vi "test_read-nmea-data2.vi"() -> ()   [LabVIEW 2019] (continued)
\t\n15:11:41.31\tF9P\t$GNGSA,A,3,12,06,19,05,17,09,04,02,,,,,1.44,0.74,1.23,1*02\n\t\n15:11:41.33\tF9P\t$GNGSA,A,3,85,71,84,,,,,,,,,,1.44,0.74,1.23,2*07\n\t\n15:11:41.35\tF9P\t$GNGSA,A,3,36,19,11,04,09,12,,,,,,,1.44,0.74,1.23,3*02\n\t\n15:11:41.37\tF9P\t$GNGSA,A,3,14,11,33,,,,,,,,,,1.44,0.74,1.23,4*03\n\t\n15:11:41.39\tF9P\t$GPGSV,3,1,09,02,54,318,23,04,18,044,22,05,37,247,25,06,64,047,32,1*6B\n\t\n15:11:41.41\tF9P\t$GPGSV,3,2,09,09,45,074,35,12,24,277,34,17,33,153,35,19,53,157,30,1*68\n\t\n15:11:41.43\tF9P\t$GPGSV,3,3,09,25,12,307,20,1*5F\n\t\n15:11:41.45\tF9P\t$GPGSV,3,1,09,02,54,318,,04,18,044,17,05,37,247,,06,64,047,23,6*6C\n\t\n15:11:41.47\tF9P\t$GPGSV,3,2,09,09,45,074,26,12,24,277,23,17,33,153,27,19,53,157,,6*6B\n\t\n15:11:41.49\tF9P\t$GPGSV,3,3,09,25,12,307,,6*5A\n\t\n15:11:41.51\tF9P\t$GLGSV,2,1,08,69,12,031,,70,71,039,,71,52,205,35,72,04,209,,1*7C\n\t\n15:11:41.53\tF9P\t$GLGSV,2,2,08,77,01,326,,84,20,122,13,85,70,065,30,86,36,330,,1*7A\n\t\n15:11:41.55\tF9P\t$GLGSV,2,1,08,69,12,031,,70,71,039,,71,52,205,25,72,04,209,,3*7F\n\t\n15:11:41.57\tF9P\t$GLGSV,2,2,08,77,01,326,,84,20,122,18,85,70,065,22,86,36,330,,3*70\n\t\n15:11:41.59\tF9P\t$GAGSV,2,1,08,02,08,297,07,04,66,118,29,09,32,193,29,11,71,358,26,7*7A\n\t\n15:11:41.61\tF9P\t$GAGSV,2,2,08,12,40,102,28,19,26,045,22,25,09,249,,36,26,308,35,7*75\n\t\n15:11:41.63\tF9P\t$GAGSV,2,1,08,02,08,297,,04,66,118,34,09,32,193,,11,71,358,,2*7B\n\t\n15:11:41.65\tF9P\t$GAGSV,2,2,08,12,40,102,,19,26,045,,25,09,249,,36,26,308,,2*7C\n\t\n15:11:41.67\tF9P\t$GBGSV,1,1,03,11,50,132,26,14,87,127,26,33,60,219,28,1*48\n\t\n15:11:41.69\tF9P\t$GBGSV,1,1,03,11,50,132,33,14,87,127,,33,60,219,,3*40\n\t\n15:11:41.71\tF9P\t$GNGLL,3723.52576,N,12656.91469,E,061143.00,A,A*75\n\t\n15:11:41.73\tF9P\t\t\n15:11:41.75\tF9P\t\t\n15:11:41.77\tF9P\t\t\n15:11:41.79\tF9P\t\t\n15:11:41.81\tF9P\t\t\n15:11:41.83\tF9P\t\t\n15:11:41.85\tF9P\t\t\n15:11:41.87\tF9P\t\t\n15:11:41.89\tF9P\t\t\n15:11:41.91\tF9P\t\t\n15:11:41.93\tF9P\t\t\n15:11:41.95\tF9P\t\t\n15:11:41.97\tF9P\t\t\n15:11:41.99\tF9P\t\t\n15:11:42.01\tF9P\t\t\n15:11:42.03\tF9P\t\t\n15:11:42.05\tF9P\t\t\n15:11:42.07\tF9P\t\t\n15:11:42.09\tF9P\t\t\n15:11:42.11\tF9P\t\t\n15:11:42.13\tF9P\t\t\n15:11:42.15\tF9P\t\t\n15:11:42.17\tF9P\t\t\n15:11:42.19\tF9P\t\t\n15:11:42.21\tF9P\t\t\n15:11:42.23\tF9P\t\t\n15:11:42.25\tF9P\t$GNRMC,061144.00,A,3723.52558,N,12656.91506,E,1.761,99.51,250720,,,A,V*3C\n\t\n15:11:42.27\tF9P\t$GNVTG,99.51,T,,M,1.761,N,3.262,K,A*13\n\t\n15:11:42.29\tF9P\t$GNGGA,061144.00,3723.52558,N,12656.91506,E,1,12,0.71,35.1,M,18.5,M,,*7D\n\t\n15:11:42.31\tF9P\t$GNGSA,A,3,12,06,19,05,17,09,04,02,,,,,1.29,0.71,1.08,1*05\n\t\n15:11:42.33\tF9P\t$GNGSA,A,3,85,71,84,,,,,,,,,,1.29,0.71,1.08,2*00\n\t\n15:11:42.35\tF9P\t$GNGSA,A,3,36,19,11,04,09,12,,,,,,,1.29,0.71,1.08,3*05\n\t\n15:11:42.37\tF9P\t$GNGSA,A,3,14,11,33,,,,,,,,,,1.29,0.71,1.08,4*04\n\t\n15:11:42.39\tF9P\t$GPGSV,3,1,09,02,54,318,26,04,18,044,22,05,37,247,25,06,64,047,31,1*6D\n\t\n15:11:42.41\tF9P\t$GPGSV,3,2,09,09,45,074,34,12,24,277,42,17,33,153,32,19,53,157,30,1*6F\n\t\n15:11:42.43\tF9P\t$GPGSV,3,3,09,25,12,307,21,1*5E\n\t\n15:11:42.45\tF9P\t$GPGSV,3,1,09,02,54,318,,04,18,044,17,05,37,247,,06,64,047,31,6*6F\n\t\n15:11:42.47\tF9P\t$GPGSV,3,2,09,09,45,074,31,12,24,277,25,17,33,153,26,19,53,157,,6*6A\n\t\n15:11:42.49\tF9P\t$GPGSV,3,3,09,25,12,307,,6*5A\n\t\n15:11:42.51\tF9P\t$GLGSV,2,1,08,69,12,031,,70,71,039,,71,52,205,37,72,04,209,,1*7E\n\t\n15:11:42.53\tF9P\t$GLGSV,2,2,08,77,01,326,,84,20,122,09,85,70,065,31,86,36,330,,1*70\n\t\n15:11:42.55\tF9P\t$GLGSV,2,1,08,69,12,031,,70,71,039,,71,52,205,26,72,04,209,,3*7C\n\t\n15:11:42.57\tF9P\t$GLGSV,2,2,08,77,01,326,,84,20,122,19,85,70,065,29,86,36,330,,3*7A\n\t\n15:11:42.59\tF9P\t$GAGSV,2,1,08,02,08,297,14,04,66,118,29,09,32,193,29,11,71,358,31,7*7E\n\t\n15:11:42.61\tF9P\t$GAGSV,2,2,08,12,40,102,32,19,26,045,22,25,09,249,,36,26,308,32,7*79\n\t\n15:11:42.63\tF9P\t$GAGSV,2,1,08,02,08,297,,04,66,118,33,09,32,193,,11,71,358,,2*7C\n\t\n15:11:42.65\tF9P\t$GAGSV,2,2,08,12,40,102,,19,26,045,,25,09,249,,36,26,308,,2*7C\n\t\n15:11:42.67\tF9P\t$GBGSV,1,1,03,11,50,132,28,14,87,127,26,33,60,219,36,1*49\n\t\n15:11:42.69\tF9P\t$GBGSV,1,1,03,11,50,132,33,14,87,127,,33,60,219,,3*40\n\t\n15:11:42.71\tF9P\t$GNGLL,3723.52558,N,12656.91506,E,061144.00,A,A*76\n\t\n15:11:42.73\tF9P\t\t\n15:11:42.75\tF9P\t\t\n15:11:42.77\tF9P\t\t\n15:11:42.79\tF9P\t\t\n15:11:42.81\tF9P\t\t\n15:11:42.83\tF9P\t\t\n15:11:42.85\tF9P\t\t\n15:11:42.87\tF9P\t\t\n15:11:42.89\tF9P\t\t\n15:11:42.91\tF9P\t\t\n15:11:42.93\tF9P\t\t\n15:11:42.95\tF9P\t\t\n15:11:42.97\tF9P\t\t\n15:11:42.99\tF9P\t\t\n15:11:43.01\tF9P\t\t\n15:11:43.03\tF9P\t\t\n15:11:43.05\tF9P\t\t\n15:11:43.07\tF9P\t\t\n15:11:43.09\tF9P\t\t\n15:11:43.11\tF9P\t\t\n15:11:43.13\tF9P\t\t\n15:11:43.15\tF9P\t\t\n15:11:43.17\tF9P\t\t\n15:11:43.19\tF9P\t\t\n15:11:43.21\tF9P\t\t\n15:11:43.23\tF9P\t\t\n15:11:43.25\tF9P\t$GNRMC,061145.00,A,3723.52534,N,12656.91513,E,1.259,108.79,250720,,,A,V*0E\n\t\n15:11:43.27\tF9P\t$GNVTG,108.79,T,,M,1.259,N,2.331,K,A*28\n\t\n15:11:43.29\tF9P\t$GNGGA,061145.00,3723.52534,N,12656.91513,E,1,12,0.71,36.9,M,18.5,M,,*79\n\t\n15:11:43.31\tF9P\t$GNGSA,A,3,12,06,19,05,17,09,04,02,,,,,1.29,0.71,1.08,1*05\n\t\n15:11:43.33\tF9P\t$GNGSA,A,3,85,71,84,,,,,,,,,,1.29,0.71,1.08,2*00\n\t\n15:11:43.35\tF9P\t$GNGSA,A,3,36,19,11,04,09,12,,,,,,,1.29,0.71,1.08,3*05\n\t\n15:11:43.37\tF9P\t$GNGSA,A,3,14,11,33,,,,,,,,,,1.29,0.71,1.08,4*04\n\t\n15:11:43.39\tF9P\t$GPGSV,3,1,09,02,54,318,34,04,18,044,22,05,37,247,25,06,64,047,27,1*69\n\t\n15:11:43.41\tF9P\t$GPGSV,3,2,09,09,45,074,36,12,24,277,42,17,33,153,38,19,53,157,29,1*6F\n\t\n15:11:43.43\tF9P\t$GPGSV,3,3,09,25,12,307,20,1*5F\n\t\n15:11:43.45\tF9P\t$GPGSV,3,1,09,02,54,318,,04,18,044,15,05,37,247,17,06,64,047,24,6*6F\n\t\n15:11:43.47\tF9P\t$GPGSV,3,2,09,09,45,074,28,12,24,277,31,17,33,153,23,19,53,157,,6*62\n\t\n15:11:43.49\tF9P\t$GPGSV,3,3,09,25,12,307,,6*5A\n\t\n15:11:43.51\tF9P\t$GLGSV,2,1,08,69,12,031,,70,71,039,,71,52,205,43,72,04,209,,1*7D\n\t\n15:11:43.53\tF9P\t$GLGSV,2,2,08,77,01,326,,84,20,122,11,85,70,065,37,86,36,330,,1*7F\n\t\n15:11:43.55\tF9P\t$GLGSV,2,1,08,69,12,031,,70,71,039,,71,52,205,25,72,04,209,,3*7F\n\t\n15:11:43.57\tF9P\t$GLGSV,2,2,08,77,01,326,,84,20,122,19,85,70,065,21,86,36,330,,3*72\n\t\n15:11:43.59\tF9P\t$GAGSV,2,1,08,02,08,297,09,04,66,118,29,09,32,193,34,11,71,358,34,7*7B\n\t\n15:11:43.61\tF9P\t$GAGSV,2,2,08,12,40,102,32,19,26,045,23,25,09,249,,36,26,308,35,7*7F\n\t\n15:11:43.63\tF9P\t$GAGSV,2,1,08,02,08,297,,04,66,118,,09,32,193,,11,71,358,,2*7C\n\t\n15:11:43.65\tF9P\t$GAGSV,2,2,08,12,40,102,,19,26,045,,25,09,249,,36,26,308,,2*7C\n\t\n15:11:43.67\tF9P\t$GBGSV,1,1,03,11,50,132,32,14,87,127,32,33,60,219,35,1*44\n\t\n15:11:43.69\tF9P\t$GBGSV,1,1,03,11,50,132,29,14,87,127,29,33,60,219,,3*40\n\t\n15:11:43.71\tF9P\t$GNGLL,3723.52534,N,12656.91513,E,061145.00,A,A*79\n\t\n15:11:43.73\tF9P\t\t\n15:11:43.75\tF9P\t\t\n15:11:43.77\tF9P\t\t\n15:11:43.79\tF9P\t\t\n15:11:43.81\tF9P\t\t\n15:11:43.83\tF9P\t\t\n15:11:43.85\tF9P\t\t\n15:11:43.87\tF9P\t\t\n15:11:43.89\tF9P\t\t\n15:11:43.91\tF9P\t\t\n15:11:43.93\tF9P\t\t\n15:11:43.95\tF9P\t\t\n15:11:43.97\tF9P\t\t\n15:11:43.99\tF9P\t\t\n15:11:44.01\tF9P\t\t\n15:11:44.03\tF9P\t\t\n15:11:44.05\tF9P\t\t\n15:11:44.07\tF9P\t\t\n15:11:44.09\tF9P\t\t\n15:11:44.11\tF9P\t\t\n15:11:44.13\tF9P\t\t\n15:11:44.15\tF9P\t\t\n15:11:44.17\tF9P\t\t\n15:11:44.19\tF9P\t\t\n15:11:44.21\tF9P\t\t\n15:11:44.23\tF9P\t\t\n15:11:44.25\tF9P\t$GNRMC,061146.00,A,3723.52516,N,12656.91546,E,1.741,93.31,250720,,,A,V*3E\n\t\n15:11:44.27\tF9P\t$GNVTG,93.31,T,,M,1.741,N,3.225,K,A*1E\n\t\n15:11:44.29\tF9P\t$GNGGA,061146.00,3723.52516,N,12656.91546,E,1,12,0.74,37.2,M,18.5,M,,*75\n\t\n15:11:44.31\tF9P\t$GNGSA,A,3,12,06,19,05,17,09,04,02,,,,,1.44,0.74,1.23,1*02\n\t\n15:11:44.33\tF9P\t$GNGSA,A,3,85,71,84,,,,,,,,,,1.44,0.74,1.23,2*07\n\t\n15:11:44.35\tF9P\t$GNGSA,A,3,36,19,11,04,09,12,,,,,,,1.44,0.74,1.23,3*02\n\t\n15:11:44.37\tF9P\t$GNGSA,A,3,14,11,33,,,,,,,,,,1.44,0.74,1.23,4*03\n\t\n15:11:44.39\tF9P\t$GPGSV,3,1,09,02,54,318,38,04,18,044,20,05,37,247,26,06,64,047,28,1*6B\n\t\n15:11:44.41\tF9P\t$GPGSV,3,2,09,09,45,074,37,12,24,277,42,17,33,153,35,19,53,157,35,1*6E\n\t\n15:11:44.43\tF9P\t$GPGSV,3,3,09,25,12,307,19,1*55\n\t\n15:11:44.45\tF9P\t$GPGSV,3,1,09,02,54,318,,04,18,044,15,05,37,247,16,06,64,047,22,6*68\n\t\n15:11:44.47\tF9P\t$GPGSV,3,2,09,09,45,074,26,12,24,277,26,17,33,153,23,19,53,157,,6*6A\n\t\n15:11:44.49\tF9P\t$GPGSV,3,3,09,25,12,307,,6*5A\n\t\n15:11:44.51\tF9P\t$GLGSV,2,1,08,69,12,031,,70,71,039,,71,52,205,40,72,04,209,,1*7E\n\t\n15:11:44.53\tF9P\t$GLGSV,2,2,08,77,01,326,,84,20,122,15,85,70,065,23,86,36,330,,1*7E\n\t\n15:11:44.55\tF9P\t$GLGSV,2,1,08,69,12,031,,70,71,039,,71,52,205,26,72,04,209,,3*7C\n\t\n15:11:44.57\tF9P\t$GLGSV,2,2,08,77,01,326,,84,20,122,20,85,70,065,29,86,36,330,,3*70\n\t\n15:11:44.59\tF9P\t$GAGSV,2,1,08,02,08,297,07,04,66,118,33,09,32,193,37,11,71,358,33,7*7A\n\t\n15:11:44.61\tF9P\t$GAGSV,2,2,08,12,40,102,36,19,26,045,21,25,09,249,,36,26,308,25,7*78\n\t\n15:11:44.63\tF9P\t$GAGSV,2,1,08,02,08,297,,04,66,118,,09,32,193,,11,71,358,,2*7C\n\t\n15:11:44.65\tF9P\t$GAGSV,2,2,08,12,40,102,,19,26,045,,25,09,249,,36,26,308,,2*7C\n\t\n15:11:44.67\tF9P\t$GBGSV,1,1,03,11,50,132,26,14,87,127,27,33,60,219,30,1*40\n\t\n15:11:44.69\tF9P\t$GBGSV,1,1,03,11,50,132,29,14,87,127,33,33,60,219,,3*4B\n\t\n15:11:44.71\tF9P\t$GNGLL,3723.52516,N,12656.91546,E,061146.00,A,A*7A\n\t\n15:11:44.73\tF9P\t\t\n15:11:44.75\tF9P\t\t\n15:11:44.77\tF9P\t\t\n15:11:44.79\tF9P\t\t\n15:11:44.81\tF9P\t\t\n15:11:44.83\tF9P\t\t\n15:11:44.85\tF9P\t\t\n15:11:44.87\tF9P\t\t\n15:11:44.89\tF9P\t\t\n15:11:44.91\tF9P\t\t\n15:11:44.93\tF9P\t\t\n15:11:44.95\tF9P\t\t\n15:11:44.97\tF9P\t\t\n15:11:44.99\tF9P\t\t\n15:11:45.01\tF9P\t\t\n15:11:45.03\tF9P\t\t\n15:11:45.05\tF9P\t\t\n15:11:45.07\tF9P\t\t\n15:11:45.09\tF9P\t\t\n15:11:45.11\tF9P\t\t\n15:11:45.13\tF9P\t\t\n15:11:45.15\tF9P\t\t\n15:11:45.17\tF9P\t\t\n15:11:45.19\tF9P\t\t\n15:11:45.21\tF9P\t\t\n15:11:45.23\tF9P\t\t\n15:11:45.25\tF9P\t$GNRMC,061147.00,A,3723.52513,N,12656.91610,E,2.332,75.44,250720,,,A,V*33\n\t\n15:11:45.27\tF9P\t$GNVTG,75.44,T,,M,2.332,N,4.320,K,A*14\n\t\n15:11:45.29\tF9P\t$GNGGA,061147.00,3723.52513,N,12656.91610,E,1,12,0.68,36.4,M,18.5,M,,*7B\n\t\n15:11:45.31\tF9P\t$GNGSA,A,3,12,06,19,05,17,09,04,02,,,,,1.27,0.68,1.08,1*03\n\t\n15:11:45.33\tF9P\t$GNGSA,A,3,85,71,84,,,,,,,,,,1.27,0.68,1.08,2*06\n\t\n15:11:45.35\tF9P\t$GNGSA,A,3,36,19,11,04,09,12,,,,,,,1.27,0.68,1.08,3*03\n\t\n15:11:45.37\tF9P\t$GNGSA,A,3,14,11,33,,,,,,,,,,1.27,0.68,1.08,4*02\n\t\n15:11:45.39\tF9P\t$GPGSV,3,1,09,02,54,318,33,04,18,044,21,05,37,247,26,06,64,047,27,1*6E\n\t\n15:11:45.41\tF9P\t$GPGSV,3,2,09,09,45,074,34,12,24,277,45,17,33,153,33,19,53,157,31,1*68\n\t\n15:11:45.43\tF9P\t$GPGSV,3,3,09,25,12,307,18,1*54\n\t\n15:11:45.45\tF9P\t$GPGSV,3,1,09,02,54,318,,04,18,044,13,05,37,247,16,06,64,047,25,6*69\n\t\n15:11:45.47\tF9P\t$GPGSV,3,2,09,09,45,074,32,12,24,277,25,17,33,153,23,19,53,157,,6*6C\n\t\n15:11:45.49\tF9P\t$GPGSV,3,3,09,25,12,307,,6*5A\n\t\n15:11:45.51\tF9P\t$GLGSV,2,1,08,69,12,031,,70,71,039,,71,52,205,44,72,04,209,,1*7A\n\t\n15:11:45.53\tF9P\t$GLGSV,2,2,08,77,01,326,,84,20,122,11,85,70,065,31,86,36,330,,1*79\n\t\n15:11:45.55\tF9P\t$GLGSV,2,1,08,69,12,031,,70,71,039,,71,52,205,26,72,04,209,,3*7C\n\t\n15:11:45.57\tF9P\t$GLGSV,2,2,08,77,01,326,,84,20,122,19,85,70,065,24,86,36,330,,3*77\n\t\n15:11:45.59\tF9P\t$GAGSV,2,1,08,02,08,297,11,04,66,118,29,09,32,193,35,11,71,358,29,7*7F\n\t\n15:11:45.61\tF9P\t$GAGSV,2,2,08,12,40,102,29,19,26,045,22,25,09,249,,36,26,308,27,7*77\n\t\n15:11:45.63\tF9P\t$GAGSV,2,1,08,02,08,297,,04,66,118,29,09,32,193,29,11,71,358,,2*7C\n\t\n15:11:45.65\tF9P\t$GAGSV,2,2,08,12,40,102,,19,26,045,,25,09,249,,36,26,308,,2*7C\n\t\n15:11:45.67\tF9P\t$GBGSV,1,1,03,11,50,132,31,14,87,127,27,33,60,219,40,1*41\n\t\n15:11:45.69\tF9P\t$GBGSV,1,1,03,11,50,132,33,14,87,127,28,33,60,219,,3*4A\n\t\n15:11:45.71\tF9P\t$GNGLL,3723.52513,N,12656.91610,E,061147.00,A,A*7E\n\t\n15:11:45.73\tF9P\t\t\n15:11:45.75\tF9P\t\t\n15:11:45.77\tF9P\t\t\n15:11:45.79\tF9P\t\t\n15:11:45.81\tF9P\t\t\n15:11:45.83\tF9P\t\t\n15:11:45.85\tF9P\t\t\n15:11:45.87\tF9P\t\t\n15:11:45.89\tF9P\t\t\n15:11:45.91\tF9P\t\t\n15:11:45.93\tF9P\t\t\n15:11:45.95\tF9P\t\t\n15:11:45.97\tF9P\t\t\n15:11:45.99\tF9P\t\t\n15:11:46.01\tF9P\t\t\n15:11:46.03\tF9P\t\t\n15:11:46.05\tF9P\t\t\n15:11:46.07\tF9P\t\t\n15:11:46.09\tF9P\t\t\n15:11:46.11\tF9P\t\t\n15:11:46.13\tF9P\t\t\n15:11:46.15\tF9P\t\t\n15:11:46.17\tF9P\t\t\n15:11:46.19\tF9P\t\t\n15:11:46.21\tF9P\t\t\n15:11:46.23\tF9P\t\t\n15:11:46.25\tF9P\t$GNRMC,061148.00,A,3723.52495,N,12656.91664,E,2.073,78.87,250720,,,A,V*34\n\t\n15:11:46.27\tF9P\t$GNVTG,78.87,T,,M,2.073,N,3.840,K,A*1A\n\t\n15:11:46.29\tF9P\t$GNGGA,061148.00,3723.52495,N,12656.91664,E,1,12,0.68,35.6,M,18.5,M,,*79\n\t\n15:11:46.31\tF9P\t$GNGSA,A,3,12,06,19,05,17,09,04,02,,,,,1.27,0.68,1.08,1*03\n\t\n15:11:46.33\tF9P\t$GNGSA,A,3,85,71,84,,,,,,,,,,1.27,0.68,1.08,2*06\n\t\n15:11:46.35\tF9P\t$GNGSA,A,3,36,19,11,04,09,12,,,,,,,1.27,0.68,1.08,3*03\n\t\n15:11:46.37\tF9P\t$GNGSA,A,3,14,11,33,,,,,,,,,,1.27,0.68,1.08,4*02\n\t\n15:11:46.39\tF9P\t$GPGSV,3,1,09,02,54,318,38,04,18,044,21,05,37,247,27,06,64,047,36,1*64\n\t\n15:11:46.41\tF9P\t$GPGSV,3,2,09,09,45,074,40,12,24,277,43,17,33,153,32,19,53,157,26,1*6A\n\t\n15:11:46.43\tF9P\t$GPGSV,3,3,09,25,12,307,18,1*54\n\t\n15:11:46.45\tF9P\t$GPGSV,3,1,09,02,54,318,,04,18,044,12,05,37,247,17,06,64,047,30,6*6D\n\t\n15:11:46.47\tF9P\t$GPGSV,3,2,09,09,45,074,27,12,24,277,25,17,33,153,24,19,53,157,,6*6F\n\t\n15:11:46.49\tF9P\t$GPGSV,3,3,09,25,12,307,,6*5A\n\t\n15:11:46.51\tF9P\t$GLGSV,2,1,08,69,12,031,,70,71,039,,71,52,205,40,72,04,209,,1*7E\n\t\n15:11:46.53\tF9P\t$GLGSV,2,2,08,77,01,326,,84,20,122,10,85,70,067,37,86,36,330,,1*7C\n\t\n15:11:46.55\tF9P\t$GLGSV,2,1,08,69,12,031,,70,71,039,,71,52,205,25,72,04,209,,3*7F\n\t\n15:11:46.57\tF9P\t$GLGSV,2,2,08,77,01,326,,84,20,122,17,85,70,067,24,86,36,330,,3*7B\n\t\n15:11:46.59\tF9P\t$GAGSV,2,1,08,02,08,297,13,04,66,118,21,09,32,193,38,11,71,358,36,7*76\n\t\n15:11:46.61\tF9P\t$GAGSV,2,2,08,12,40,102,30,19,26,045,23,25,09,249,,36,26,308,26,7*7F\n\t\n15:11:46.63\tF9P\t$GAGSV,2,1,08,02,08,297,,04,66,118,,09,32,193,30,11,71,358,,2*7F\n\t\n15:11:46.65\tF9P\t$GAGSV,2,2,08,12,40,102,,19,26,045,,25,09,249,,36,26,308,,2*7C\n\t\n15:11:46.67\tF9P\t$GBGSV,1,1,03,11,50,132,31,14,87,127,28,33,60,219,27,1*4F\n\t\n15:11:46.69\tF9P\t$GBGSV,1,1,03,11,50,132,27,14,87,127,33,33,60,219,,3*45\n\t\n15:11:46.71\tF9P\t$GNGLL,3723.52495,N,12656.91664,E,061148.00,A,A*7D\n\t\n15:11:46.73\tF9P\t\t\n15:11:46.75\tF9P\t\t\n15:11:46.77\tF9P\t\t\n15:11:46.79\tF9P\t\t\n15:11:46.81\tF9P\t\t\n15:11:46.83\tF9P\t\t\n15:11:46.85\tF9P\t\t\n15:11:46.87\tF9P\t\t\n15:11:46.89\tF9P\t\t\n15:11:46.91\tF9P\t\t\n15:11:46.93\tF9P\t\t\n15:11:46.95\tF9P\t\t\n15:11:46.97\tF9P\t\t\n15:11:46.99\tF9P\t\t\n15:11:47.01\tF9P\t\t\n15:11:47.03\tF9P\t\t\n15:11:47.05\tF9P\t\t\n15:11:47.07\tF9P\t\t\n15:11:47.09\tF9P\t\t\n15:11:47.11\tF9P\t\t\n15:11:47.13\tF9P\t\t\n15:11:47.15\tF9P\t\t\n15:11:47.17\tF9P\t\t\n15:11:47.19\tF9P\t\t\n15:11:47.21\tF9P\t\t\n15:11:47.23\tF9P\t\t\n15:11:47.25\tF9P\t$GNRMC,061149.00,A,3723.52506,N,12656.91714,E,2.154,65.52,250720,,,A,V*38\n\t\n15:11:47.27\tF9P\t$GNVTG,65.52,T,,M,2.154,N,3.989,K,A*1E\n\t\n15:11:47.29\tF9P\t$GNGGA,061149.00,3723.52506,N,12656.91714,E,1,12,0.71,35.5,M,18.5,M,,*7E\n\t\n15:11:47.31\tF9P\t$GNGSA,A,3,12,06,19,05,17,09,04,02,,,,,1.42,0.71,1.23,1*01\n\t\n15:11:47.33\tF9P\t$GNGSA,A,3,85,71,84,,,,,,,,,,1.42,0.71,1.23,2*04\n\t\n15:11:47.35\tF9P\t$GNGSA,A,3,36,19,11,04,09,12,,,,,,,1.42,0.71,1.23,3*01\n\t\n15:11:47.37\tF9P\t$GNGSA,A,3,14,11,33,,,,,,,,,,1.42,0.71,1.23,4*00\n\t\n15:11:47.39\tF9P\t$GPGSV,3,1,09,02,54,318,39,04,18,044,22,05,37,247,26,06,64,047,36,1*67\n\t\n15:11:47.41\tF9P\t$GPGSV,3,2,09,09,45,074,30,12,24,277,36,17,33,153,30,19,53,157,34,1*6E\n\t\n15:11:47.43\tF9P\t$GPGSV,3,3,09,25,12,307,17,1*5B\n\t\n15:11:47.45\tF9P\t$GPGSV,3,1,09,02,54,318,,04,18,044,10,05,37,247,16,06,64,047,29,6*66\n\t\n15:11:47.47\tF9P\t$GPGSV,3,2,09,09,45,074,28,12,24,277,23,17,33,153,24,19,53,157,,6*66\n\t\n15:11:47.49\tF9P\t$GPGSV,3,3,09,25,12,307,,6*5A\n\t\n15:11:47.51\tF9P\t$GLGSV,2,1,08,69,12,031,,70,71,039,34,71,52,205,41,72,04,209,,1*78\n\t\n15:11:47.53\tF9P\t$GLGSV,2,2,08,77,01,326,,84,20,122,10,85,70,067,39,86,37,330,,1*73\n\t\n15:11:47.55\tF9P\t$GLGSV,2,1,08,69,12,031,,70,71,039,,71,52,205,26,72,04,209,,3*7C\n\t\n15:11:47.57\tF9P\t$GLGSV,2,2,08,77,01,326,,84,20,122,14,85,70,067,22,86,37,330,,3*7F\n\t\n15:11:47.59\tF9P\t$GAGSV,2,1,08,02,08,297,11,04,66,118,29,09,32,193,42,11,71,358,30,7*77\n\t\n15:11:47.61\tF9P\t$GAGSV,2,2,08,12,40,102,30,19,26,045,27,25,09,249,,36,26,308,26,7*7B\n\t\n15:11:47.63\tF9P\t$GAGSV,2,1,08,02,08,297,,04,66,118,,09,32,193,34,11,71,358,,2*7B\n\t\n15:11:47.65\tF9P\t$GAGSV,2,2,08,12,40,102,,19,26,045,,25,09,249,,36,26,308,,2*7C\n\t\n15:11:47.67\tF9P\t$GBGSV,1,1,03,11,50,132,31,14,87,127,29,33,60,219,35,1*4D\n\t\n15:11:47.69\tF9P\t$GBGSV,1,1,03,11,50,132,32,14,87,127,29,33,60,219,,3*4A\n\t\n15:11:47.71\tF9P\t$GNGLL,3723.52506,N,12656.91714,E,061149.00,A,A*71\n\t\n15:11:47.73\tF9P\t\t\n15:11:47.75\tF9P\t\t\n15:11:47.77\tF9P\t\t\n15:11:47.79\tF9P\t\t\n15:11:47.81\tF9P\t\t\n15:11:47.83\tF9P\t\t\n15:11:47.85\tF9P\t\t\n15:11:47.87\tF9P\t\t\n15:11:47.89\tF9P\t\t\n15:11:47.91\tF9P\t\t\n15:11:47.93\tF9P\t\t\n15:11:47.95\tF9P\t\t\n15:11:47.97\tF9P\t\t\n15:11:47.99\tF9P\t\t\n15:11:48.01\tF9P\t\t\n15:11:48.03\tF9P\t\t\n15:11:48.05\tF9P\t\t\n15:11:48.07\tF9P\t\t\n15:11:48.09\tF9P\t\t\n15:11:48.11\tF9P\t\t\n15:11:48.13\tF9P\t\t\n15:11:48.15\tF9P\t\t\n15:11:48.17\tF9P\t\t\n15:11:48.19\tF9P\t\t\n15:11:48.21\tF9P\t\t\n15:11:48.23\tF9P\t\t\n15:11:48.25\tF9P\t$GNRMC,061150.00,A,3723.52536,N,12656.91751,E,2.402,52.26,250720,,,A,V*33\n\t\n15:11:48.27\tF9P\t$GNVTG,52.26,T,,M,2.402,N,4.449,K,A*19\n\t\n15:11:48.29\tF9P\t$GNGGA,061150.00,3723.52536,N,12656.91751,E,1,12,0.68,35.5,M,18.5,M,,*7C\n\t\n15:11:48.31\tF9P\t$GNGSA,A,3,12,06,19,05,17,09,04,02,,,,,1.27,0.68,1.08,1*03\n\t\n15:11:48.33\tF9P\t$GNGSA,A,3,85,71,84,,,,,,,,,,1.27,0.68,1.08,2*06\n\t\n15:11:48.35\tF9P\t$GNGSA,A,3,36,19,11,04,09,12,,,,,,,1.27,0.68,1.08,3*03\n\t\n15:11:48.37\tF9P\t$GNGSA,A,3,14,11,33,,,,,,,,,,1.27,0.68,1.08,4*02\n\t\n15:11:48.39\tF9P\t$GPGSV,3,1,09,02,54,318,39,04,18,044,21,05,37,247,26,06,64,047,33,1*61\n\t\n15:11:48.41\tF9P\t$GPGSV,3,2,09,09,45,074,30,12,24,277,37,17,33,153,32,19,53,157,32,1*6B\n\t\n15:11:48.43\tF9P\t$GPGSV,3,3,09,25,12,307,17,1*5B\n\t\n15:11:48.45\tF9P\t$GPGSV,3,1,09,02,54,318,,04,18,044,12,05,37,247,16,06,64,047,27,6*6A\n\t\n15:11:48.47\tF9P\t$GPGSV,3,2,09,09,45,074,20,12,24,277,23,17,33,153,24,19,53,157,,6*6E\n\t\n15:11:48.49\tF9P\t$GPGSV,3,3,09,25,12,307,,6*5A\n\t\n15:11:48.51\tF9P\t$GLGSV,2,1,08,69,12,031,,70,71,039,,71,52,205,43,72,04,209,,1*7D\n\t\n15:11:48.53\tF9P\t$GLGSV,2,2,08,77,01,326,,84,20,122,13,85,70,067,40,86,37,330,,1*7E\n\t\n15:11:48.55\tF9P\t$GLGSV,2,1,08,69,12,031,,70,71,039,,71,52,205,30,72,04,209,,3*7B\n\t\n15:11:48.57\tF9P\t$GLGSV,2,2,08,77,01,326,,84,20,122,15,85,70,067,21,86,37,330,,3*7D\n\t\n15:11:48.59\tF9P\t$GAGSV,2,1,08,02,08,297,09,04,66,118,28,09,32,193,39,11,71,358,32,7*71\n\t\n15:11:48.61\tF9P\t$GAGSV,2,2,08,12,40,102,29,19,26,045,27,25,09,249,,36,26,308,35,7*71\n\t\n15:11:48.63\tF9P\t$GAGSV,2,1,08,02,08,297,,04,66,118,,09,32,193,35,11,71,358,,2*7A\n\t\n15:11:48.65\tF9P\t$GAGSV,2,2,08,12,40,102,,19,26,045,,25,09,249,,36,26,308,,2*7C\n\t\n15:11:48.67\tF9P\t$GBGSV,1,1,03,11,50,132,26,14,87,127,33,33,60,219,39,1*4C\n\t\n15:11:48.69\tF9P\t$GBGSV,1,1,03,11,50,132,29,14,87,127,32,33,60,219,,3*4A\n\t\n15:11:48.71\tF9P\t$GNGLL,3723.52536,N,12656.91751,E,061150.00,A,A*7B\n\t\n15:11:48.73\tF9P\t\t\n15:11:48.75\tF9P\t\t\n15:11:48.77\tF9P\t\t\n15:11:48.79\tF9P\t\t\n15:11:48.81\tF9P\t\t\n15:11:48.83\tF9P\t\t\n15:11:48.85\tF9P\t\t\n15:11:48.87\tF9P\t\t\n15:11:48.89\tF9P\t\t\n15:11:48.91\tF9P\t\t\n15:11:48.93\tF9P\t\t\n15:11:48.95\tF9P\t\t\n15:11:48.97\tF9P\t\t\n15:11:48.99\tF9P\t\t\n15:11:49.01\tF9P\t\t\n15:11:49.03
